vi "VD-getData.vi"(8 "error in (no error)":errorcluster, 10 "data req":T2, 11 "VD-LV-LiteVNA in":refnum<class "VD-LV-LiteVNA.lvclass">) -> (0 "error out":errorcluster, 2 "read buffer":T1 format="%x", 3 "VD-LV-LiteVNA out":refnum<class "VD-LV-LiteVNA.lvclass">)   [LabVIEW 2020, in "VD-LV-LiteVNA.lvclass"]
uses:
  VD-LV-LiteVNA.lvclass
  VD-data_req.ctl
  hardware-protocol/serial/HP-S-data.ctl
  VD-action.ctl
  VD-LV-LiteVNA.lvclass/VD-LV-LiteVNA.ctl
  hardware-protocol/serial/HP-S-Serial.lvclass
panel:
  out "ms":u32
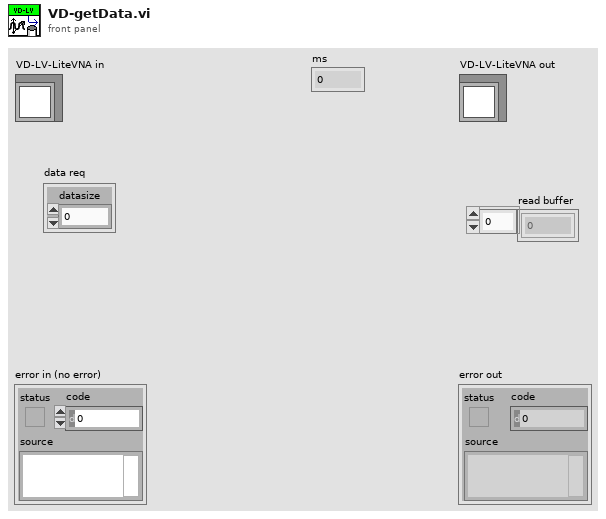
[diagram p1: front panel]
types:
  T1 = typedef "HP-S-Serial.lvclass/HP-S-data.ctl" = u8[]
  T2 = typedef "VD-LV-LiteVNA.lvclass/VD-data_req.ctl" = cluster{"datasize":u8}
  T3 = typedef "VD-LV-LiteVNA.lvclass/VD-action.ctl" = enum16{"checkCom", "SweepStartHz", "SweepStopHz", "SweepPoints", "valuesPerFrequency", "RawSamplesMode", "ValuesFIFO", "deviceVariant", "protocolVersion", "hardwareRevision", "firmwareMajor", "firmwareMinor"}
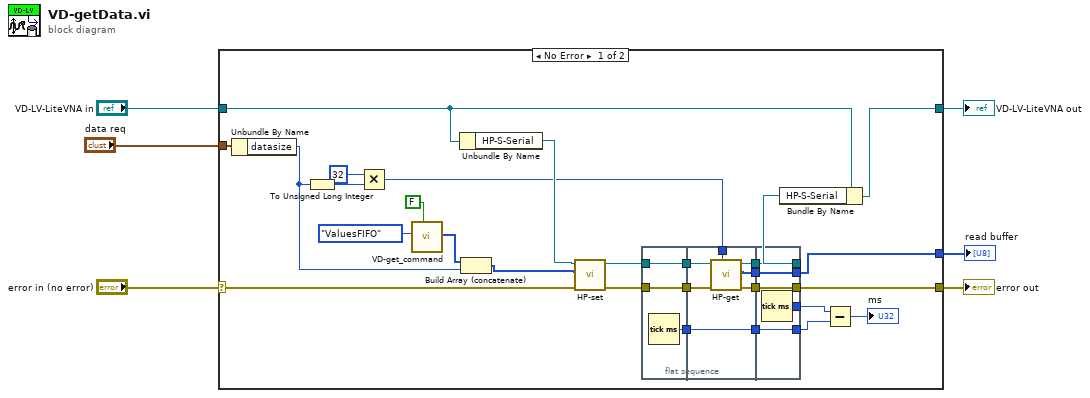
[diagram p0: block diagram]
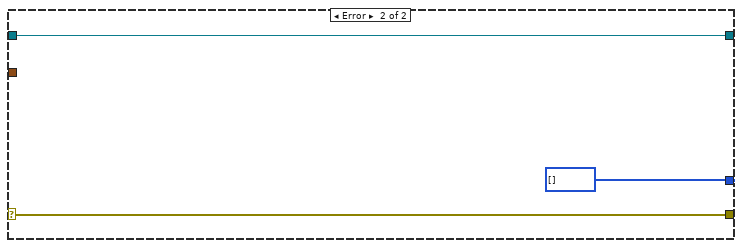
[diagram p2: hidden frame]
diagram:
  n1 = case shown="No Error" "error in (no error)" {
    selector: "error in (no error)" -> [w26 w52]
    tunnel: [w22 w52] -> w5
    tunnel: [w33 w51] -> w3
    tunnel: "VD-LV-LiteVNA in" -> [w34 w51]
    tunnel: "data req" -> [w32 _]
    tunnel: [w7 T1 [] ("read buffer")] -> w1
    frame No Error {
      n2 = Unbundle By Name(w32) -> ("datasize"=w21:u8)
      n3 = To Unsigned Long Integer(number=w21) -> (unsigned 32bit integer=w18:u32)
      n4 = Multiply(x=u32 32, y=w18) -> (x*y=w19:u32)
      n5 = call "VD-get_command.vi"("Write?"=FALSE, "action"=VD-action."ValuesFIFO") -> ("Command"=w31:T1)  [unwired: 9 in]
      n6 = Unbundle By Name(w34) -> ("HP-S-Serial"=w28:refnum<class "HP-S-Serial.lvclass">)
      n7 = Build Array (concatenate)(w31, w21) -> (w27:T1)
      n8 = call-dynamic "HP-set.vi"("error in (no error)"=w26, "write buffer"=w27, "HP-S-Serial in"=w28) -> ("error out"=w25:errorcluster, "HP-S-Serial out"=w24:refnum<class "HP-S-Serial.lvclass">)  [unwired: 7 in]
      n9 = flat-sequence {
        tunnel: w24 -> [w36]
        tunnel: w25 -> [w37]
        tunnel: [w37] -> w14
        tunnel: [w36] -> w13
        tunnel: [w35] -> w11
        tunnel: w19 -> [w39]
        tunnel: [w42] -> w17
        tunnel: [w41] -> w16
        tunnel: [w40] -> w15
        tunnel: w14 -> [w44]
        tunnel: w13 -> [w43]
        tunnel: [w38] -> w12
        tunnel: w11 -> [w38]
        tunnel: [w47] -> w22
        tunnel: [w48] -> w7
        tunnel: [w49] -> w23
        tunnel: w17 -> [w49]
        tunnel: w16 -> [w48]
        tunnel: w15 -> [w47]
        tunnel: w12 -> [w45]
        tunnel: [w46] -> w9
        tunnel: [w45] -> w10
        frame #0 {
          n10 = Tick Count (ms)() -> (millisecond timer value=w35:u32)
        }
        frame #1 {
          n11 = call-dynamic "HP-get.vi"("get byte count"=w39, "error in (no error)"=w44, "HP-S-Serial in"=w43) -> ("error out"=w40:errorcluster, "read buffer"=w41:T1, "HP-S-Serial out"=w42:refnum<class "HP-S-Serial.lvclass">)  [unwired: 6 in]
        }
        frame #2 {
          n12 = Tick Count (ms)() -> (millisecond timer value=w46:u32)
        }
      }
      n13 = Bundle By Name(cluster=w34, "HP-S-Serial"=w23) -> (w33:refnum<class "VD-LV-LiteVNA.lvclass">)
      n14 = Subtract(x=w9, y=w10) -> (x-y=→"ms":u32)
    }
    frame Error {
    }
  }
  "error out" <- w5
  "VD-LV-LiteVNA out" <- w3
  "read buffer" <- w1
